vi "Parse MISO Signal.vi"(7 "SPI Configuration":T1={"CLK Frequency (Hz)"=250000, "CPOL"=FALSE, "CPHA"=FALSE, "CS Channel"="", "CLK Channel"="", "MOSI Channel"="", "MISO Channel"="", "Active CS"=FALSE, "Dig In Task"="", "Dig Out Task"=""} {"CLK Frequency (Hz)" format="%#.6p"}, 8 "Error In":errorcluster, 11 "SPI Signals":digitalwaveform(waveform)={"t0"=timestamp(0 s since 1904-01-01), "dt"=0.0, "Y"={"transitions"=[], "data"=[]}, "error"={"status"=FALSE, "code"=37421928, "source"=""}}) -> (0 "Error Out":errorcluster, 3 "MISO Data":u8[](array[numeric]) format="%x")   [LabVIEW 2016, in "SPIVI.lvlib"]
uses:
  SPIVI.lvlib
  Typedefs/SPI Configuration.ctl
  <vilib>/Waveform/DWDTOps.llb/DWDT Digital to Boolean Array.vi
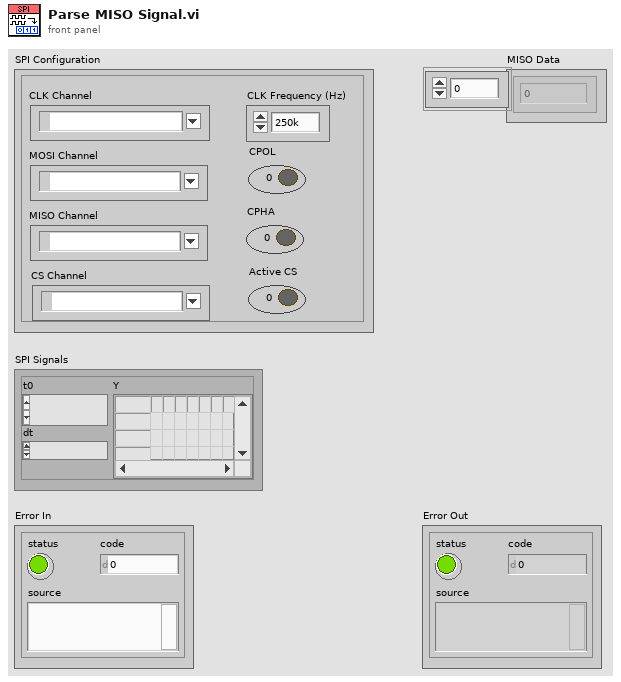
[diagram p1: front panel]
types:
  T1 = typedef "SPIVI.lvlib/SPI Configuration.ctl" = cluster{"CLK Frequency (Hz)":u32, "CPOL":bool, "CPHA":bool, "CS Channel":tag, "CLK Channel":tag, "MOSI Channel":tag, "MISO Channel":tag, "Active CS":bool, "Dig In Task":refnum<k21>, "Dig Out Task":refnum<k21>}
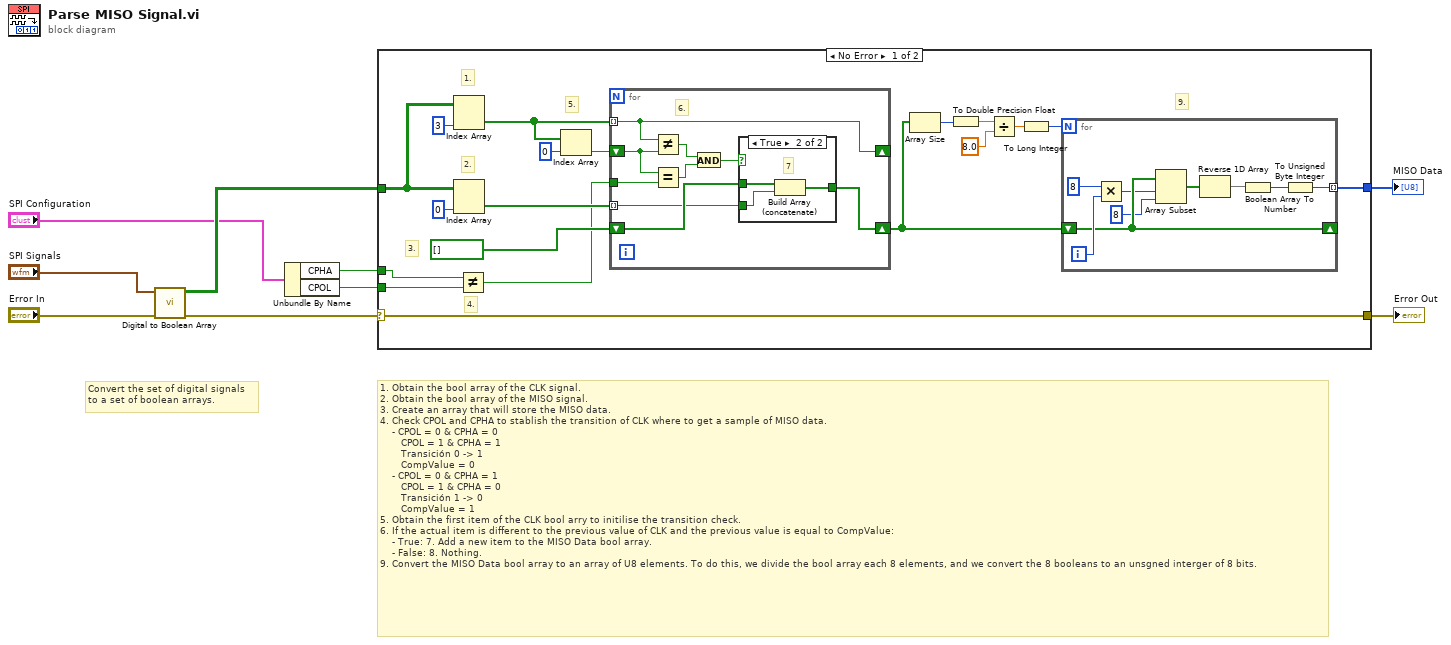
[diagram p0: block diagram]
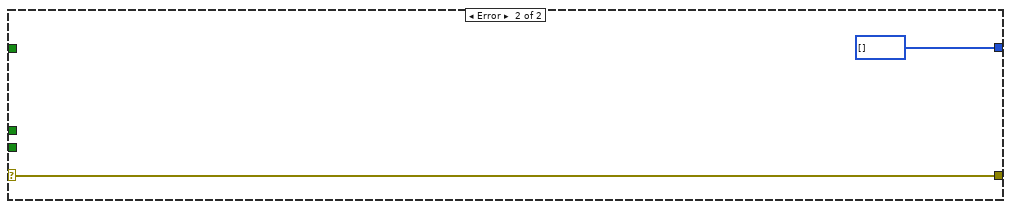
[diagram p3: hidden frame]
diagram:
  # "Convert the set of digital signals\nto a set of boolean arrays."
  # "1. Obtain the bool array of the CLK signal.\n2. Obtain the bool array of the MISO signal.\n3. Create an array that will store the MISO data.\n4. Check CPOL and CPHA to stablish the transition of CLK where to get a sample of MISO data.\n    - CPOL = 0 & CPHA = 0\n       CPOL = 1 & CPHA = 1\n       Transición 0 -> 1\n       CompValue = 0\n    - CPOL = 0 & CPHA = 1\n       CPOL = 1 & CPHA = 0\n       Transición 1 -> 0\n       CompValue = 1\n5. Obtain the first item of the CLK bool arry to initilise the transition check.\n6. If the actual item is different to the previous value of CLK and the previous value is equal to CompValue:\n    - True: 7. Add a new item to the MISO Data bool array.\n    - False: 8. Nothing.\n9. Convert the MISO Data bool array to an array of U8 elements. To do this, we divide the bool array each 8 elements, and we convert the 8 booleans to an unsgned interger of 8 bits."
  n1 = call-poly <vilib>:"Digital to Boolean Array.vi"("error in (no error)"="Error In", "digital waveform"="SPI Signals") -> ("error out"=w9:errorcluster, "boolean array"=w8:bool[][])  [unwired: 8 in]
  n2 = Unbundle By Name("SPI Configuration") -> ("CPHA"=w5:bool, "CPOL"=w4:bool)
  n3 = case shown="No Error" w9 {
    selector: w9 -> [w21 w52]
    tunnel: w8 -> [w26 _]
    tunnel: w4 -> [w25 _]
    tunnel: w5 -> [w10 _]
    tunnel: [w21 w52] -> w7
    tunnel: [w11 u8[] []] -> w6
    frame No Error {
      # "9."
      # "5."
      # "4."
      # "3."
      # "2."
      # "1."
      n4 = Index Array(array=w26, index (col)=3 ("disabled index (col)")) -> (element=w24:bool[])  [unwired: 1 in]
      n5 = Index Array(array=w26, index (col)=0 ("disabled index (col)")) -> (element=w22:bool[])  [unwired: 1 in]
      n6 = Not Equal?(x=w10, y=w25) -> (x != y?=w18:bool)
      n7 = Index Array(array=w24, index=0) -> (element=w19:bool)
      n8 = for {
        tunnel: w24 -> [w45] mode=indexing
        shift-right: [w45] -> _
        shift-left: w19 -> [w46]
        shift-right: [w39] -> w17
        shift-left: bool[] [] -> [w41]
        tunnel: w22 -> [w40] mode=indexing
        tunnel: w18 -> [w38]
        # "6."
        n9 = Not Equal?(x=w45, y=w46) -> (x != y?=w44:bool)
        n10 = Equal?(x=w46, y=w38) -> (x = y?=w43:bool)
        n11 = And(x=w44, y=w43) -> (x .and. y?=w42:bool)
        n12 = case shown="True" w42 {
          tunnel: w41 -> [w47 w50]
          tunnel: w40 -> [_ w49]
          tunnel: [w47 w48] -> w39
          frame False {
            # "8."
          }
          frame True {
            # "7"
            n13 = Build Array (concatenate)(w50, w49) -> (w48:bool[])
          }
        }
      }
      n14 = Array Size(array=w17) -> (size(s)=w16:i32)
      n15 = To Double Precision Float(number=w16) -> (double precision float=w12:dbl)
      n16 = Divide(x=w12, y=8.0) -> (x/y=w14:dbl)
      n17 = To Long Integer(number=w14) -> (32bit integer=w13:i32)
      n18 = for {
        N: w13 -> [_]
        shift-right: [w35] -> _
        shift-left: w17 -> [w35]
        tunnel: [w30] -> w11 mode=indexing
        i -> [w37]
        n19 = Multiply(x=8, y=w37) -> (x*y=w33:i32)
        n20 = Array Subset(array=w35, index=w33, length=8) -> (w32:bool[])
        n21 = Reverse 1D Array(array=w32) -> (reversed array=w29:bool[])
        n22 = Boolean Array To Number(Boolean array=w29) -> (number=w31:u32)
        n23 = To Unsigned Byte Integer(number=w31) -> (unsigned 8bit integer=w30:u8)
      }
    }
    frame Error {
    }
  }
  "Error Out" <- w7
  "MISO Data" <- w6
